vi "AVI_Tools.vi"() -> ()   [LabVIEW 2022 SP3]
uses:
  <vilib>/vision/Image Controls.llb/IMAQ Image.ctl
  <vilib>/vision/Avi.llb/IMAQ AVI2 Refnum.ctl
  <vilib>/vision/Avi.llb/IMAQ AVI2 Codec Path.ctl
panel:
  out "Array 2":i32[][](array[numeric])
  out "file name":string
  out "FinalImge":i32[](array[numeric])
  out "Crop Size":i32[](array[numeric])=[50, 60, 520, 360]
  in  "Tab Control":enum32{"Crop", "Output"}(tab)
  out "ref Fram":T1(plugin-control)
  in  "Crop":bool
  in  "Insertion Point":bool
  out "Output":T1(plugin-control)
  in  "Start SpliceFrame":i32=1000
  in  "#Frame":i32=260
  out "Frame":i32
  in  "Splice":u16(ring)=17 items=["Bmode CD"=17, "VPI"=26]
  out "CurrentSaveFile":string
  in  "Text Splice":u16(ring) items=["SelectText", "WT", "KO"]
  in  "Add text":string
  in  "DownSamp":u32=2
  in  "Group":i32=2
  in  "Scale":sgl
  in  "Codec Source":T2 items=["Default", "System", "Built in Vision"]
  in  "AVI save name":string
  out "Frames":u32[](array[numeric])
  out "Text Insertion Point":i32[](array[numeric])=[40, 20]
  in  "Enum":T3(ring)
  out "Array":T4(array[cluster])
  in  "Use Selected Files":bool
  in  "Listbox":i32[](listbox)
  in  "AviReadDirectory":path=path "D:/"
  in  "search pattern":string="*.avi"
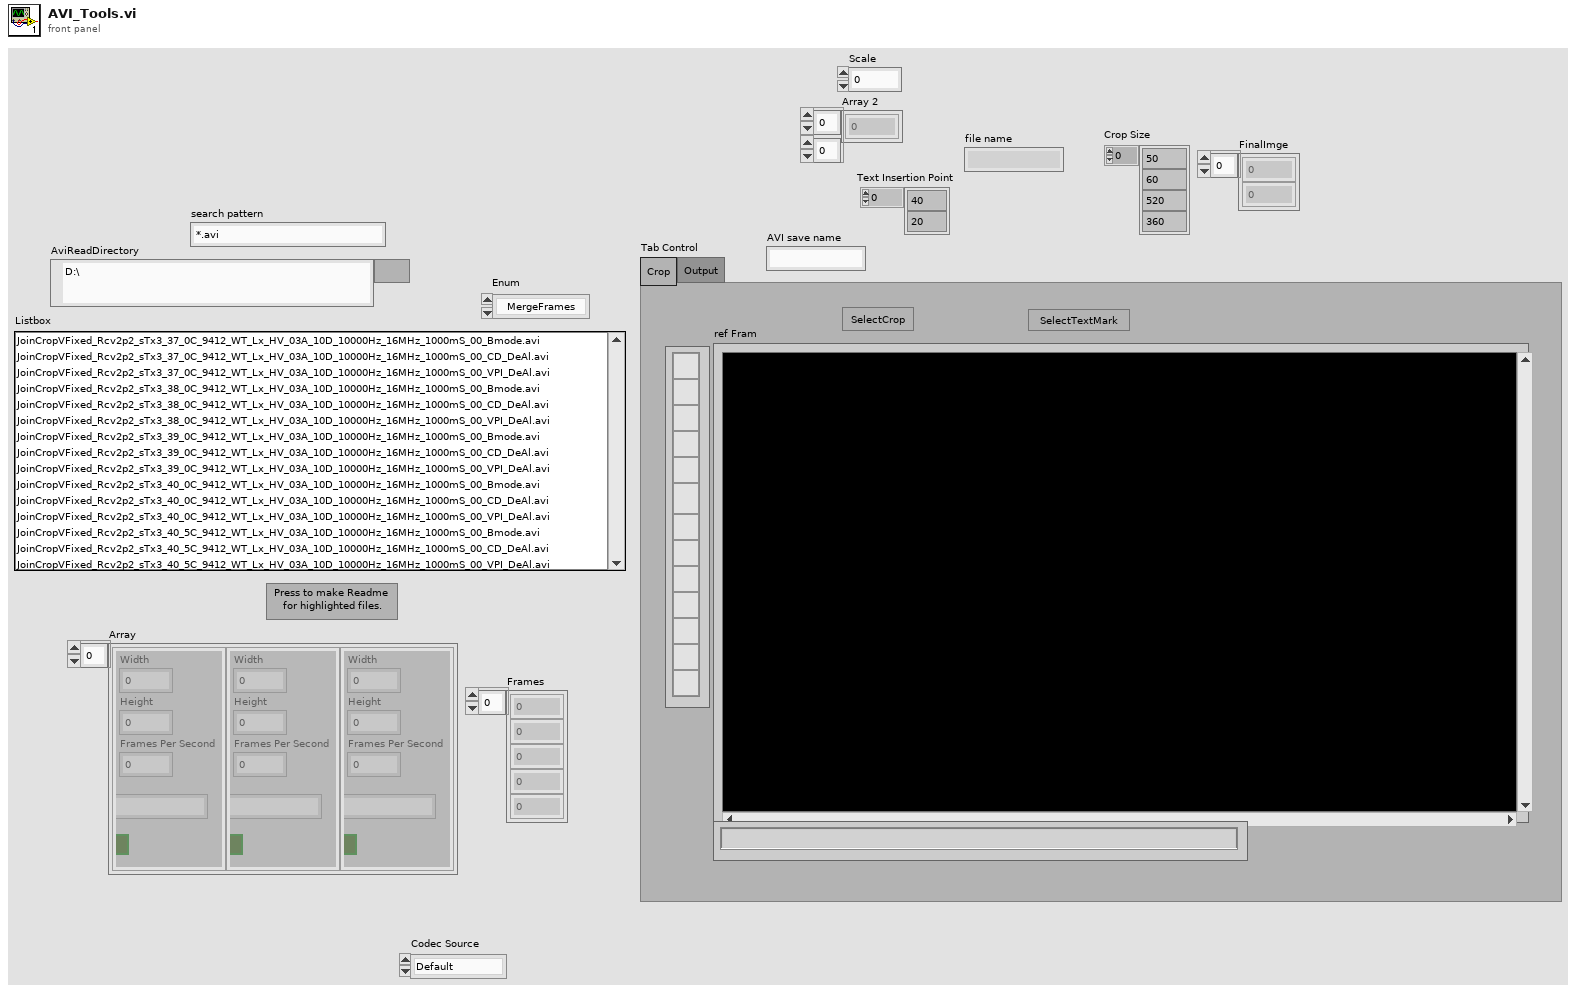
[diagram p1: front panel]
types:
  T1 = typedef "IMAQ Image.ctl" = refnum<image>
  T2 = typedef "IMAQ AVI2 Codec Path.ctl" = u32
  T3 = enum16{"MergeFrames", "Join AVI", "Crop", "OverlayText", "RescaleScale", "SpliceIn", "DownSample", "Extract"}
  T4 = cluster{"Width":u32, "Height":u32, "Frames Per Second":u32, "Codec":string, "Has Data":bool}[]
  T5 = typedef "IMAQ AVI2 Refnum.ctl" = refnum<k20>
  T6 = cluster{"Number of Frames":u32, "Frame Data":cluster{"Width":u32, "Height":u32, "Frames Per Second":u32, "Codec":string, "Has Data":bool}, "New Image":T1, "AVI Refnum":T5, "file name":string}
  T7 = typedef "Image Type" = u32
  T8 = cluster{"Width":u32, "Height":u32, "Frames Per Second":u32, "Codec":string, "Has Data":bool}
  T9 = cluster{"Desired Font (Application)":enum16{"User-specified Font", "Application Font", "System Font", "Dialog Font"}, "[User-specified Font]":cluster{"Font Name":string, "Size":i16, "Strikeout?":bool, "Italic?":bool, "Underline?":bool, "Outline?":bool, "Shadow?":bool, "Bold?":bool, "Rotation Angle":dbl}, "Horizontal Alignment":i16, "Vertical Alignment":i16}
  T10 = cluster{"Global Rectangle":i32[], "Contours":cluster{"Contour Type":u32, "ROI Type":u32, "Points":i32[]}[]}
  T11 = cluster{"Number of Frames":u32, "Frame Data":cluster{"Width":u32, "Height":u32, "Frames Per Second":u32, "Codec":string, "Has Data":bool}, "New Image":T1, "AVI Refnum":T5, "file name":string}[][]
  T12 = cluster{"Number of Frames":u32, "Frame Data":cluster{"Width":u32, "Height":u32, "Frames Per Second":u32, "Codec":string, "Has Data":bool}, "New Image":T1, "AVI Refnum":T5, "file name":string}[]
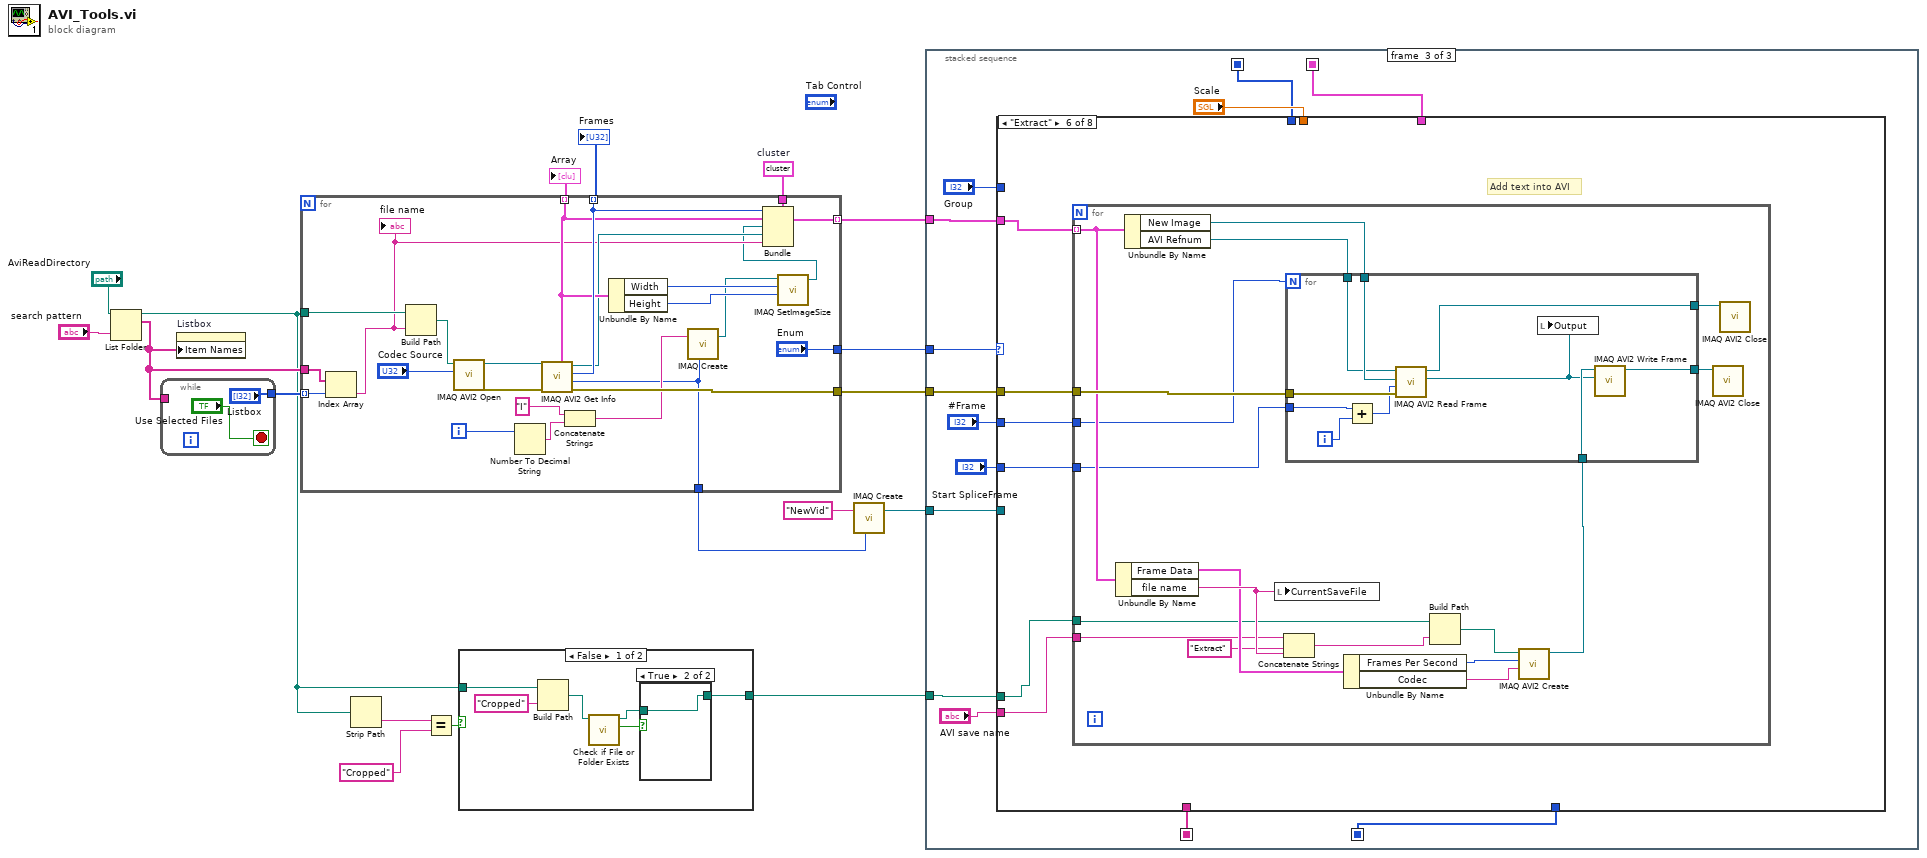
[diagram p0: block diagram]
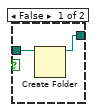
[diagram p2: hidden frame]
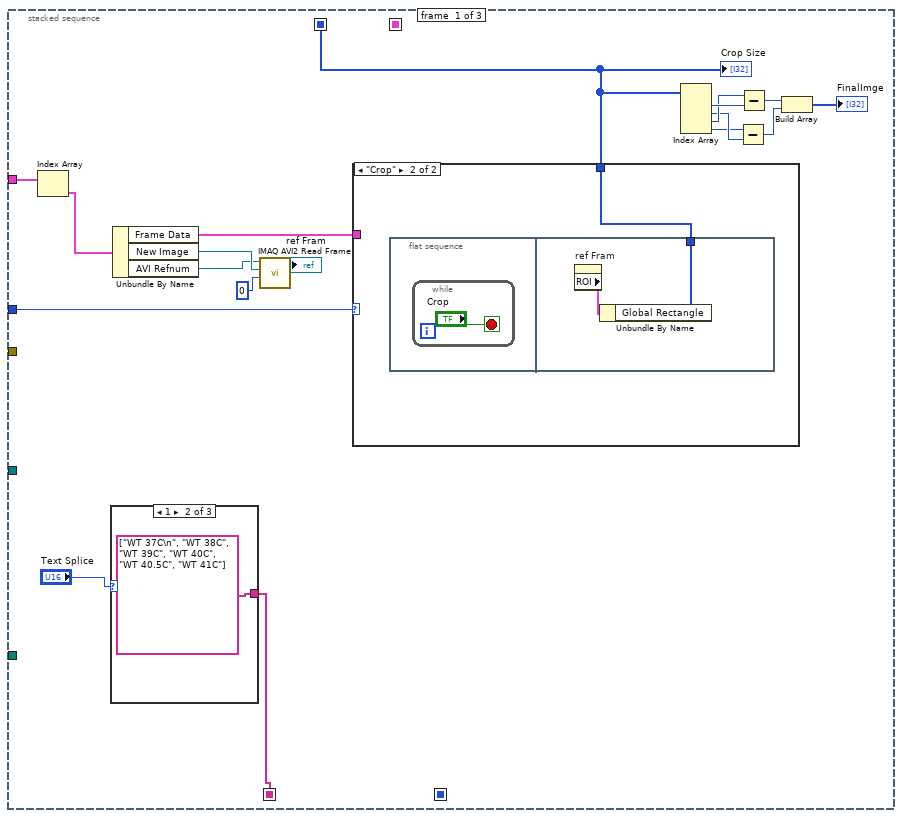
[diagram p4: hidden frame]
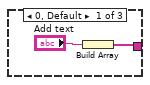
[diagram p5: hidden frame]
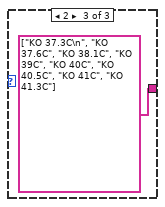
[diagram p6: hidden frame]
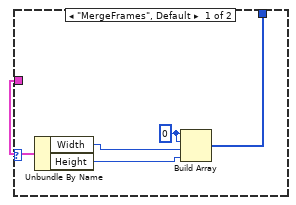
[diagram p7: hidden frame]
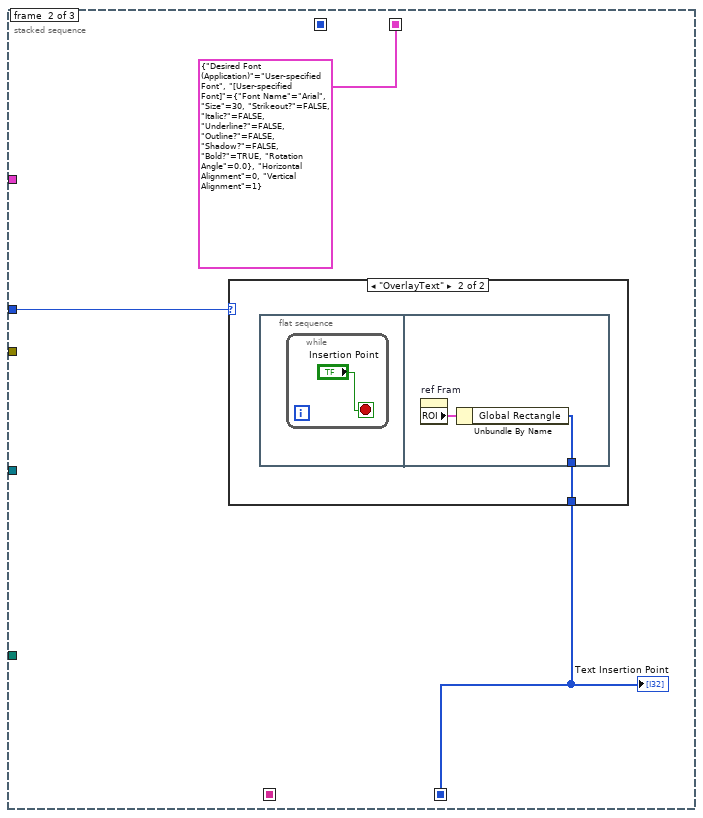
[diagram p8: hidden frame]
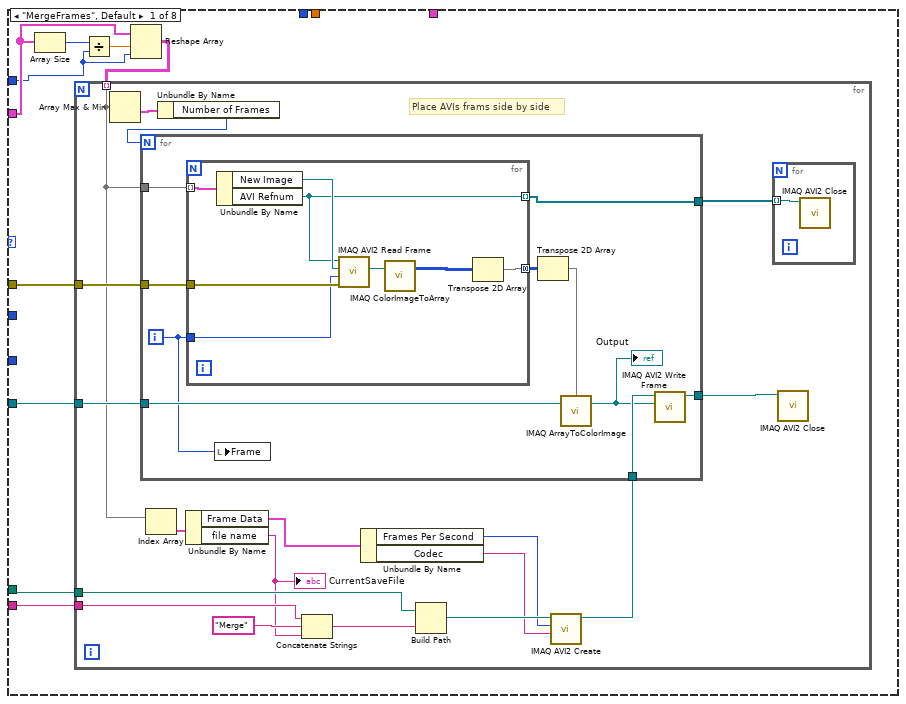
[diagram p10: hidden frame]
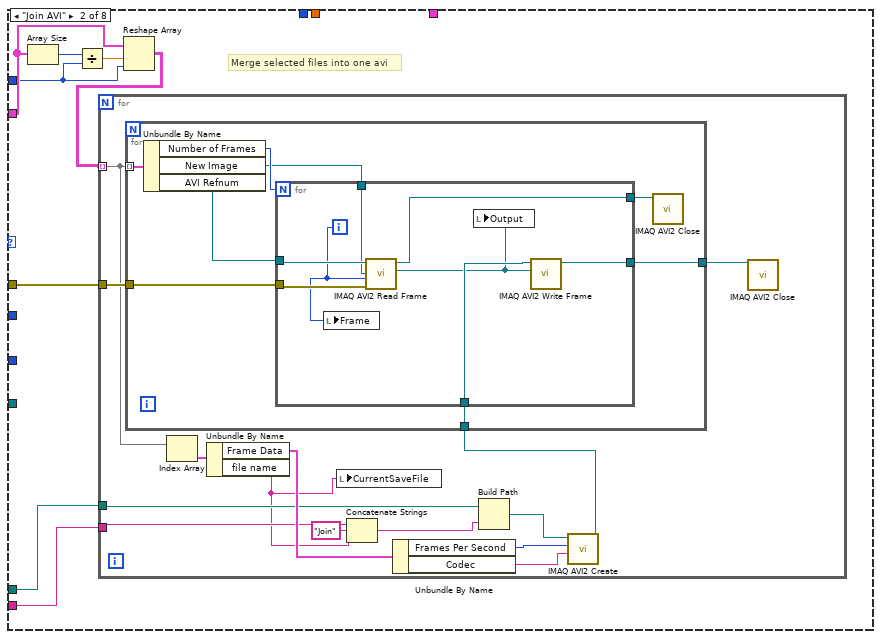
[diagram p11: hidden frame]
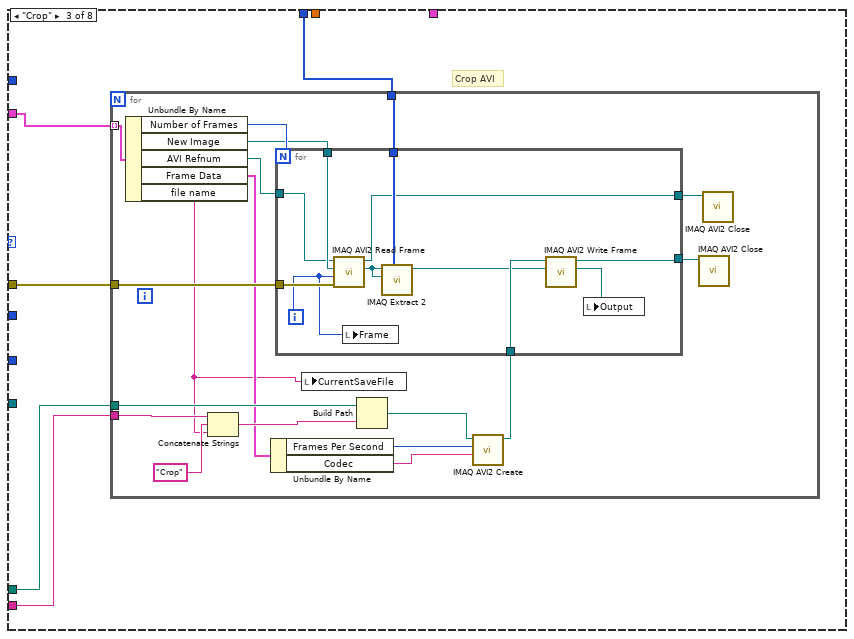
[diagram p12: hidden frame]
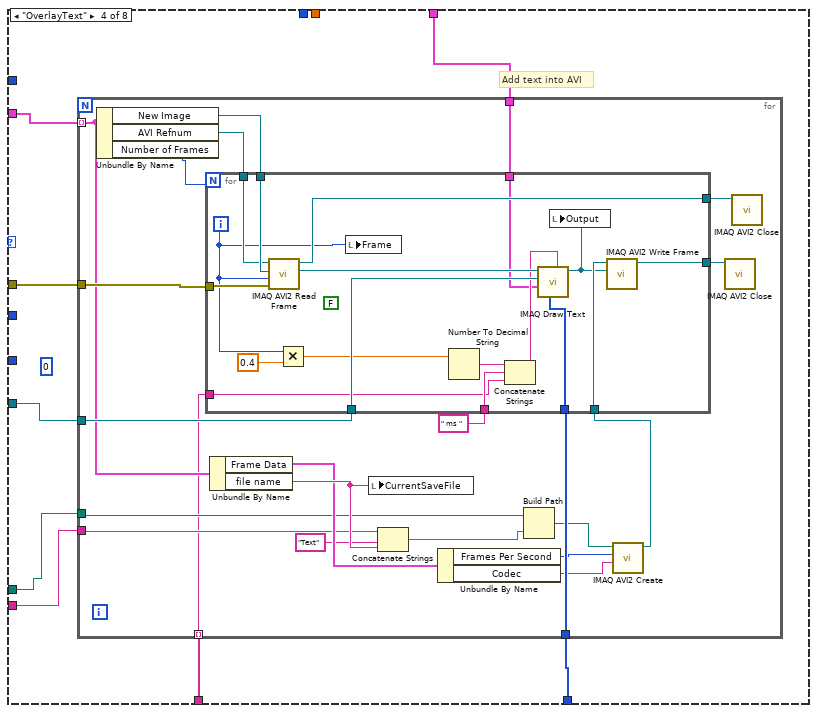
[diagram p13: hidden frame]
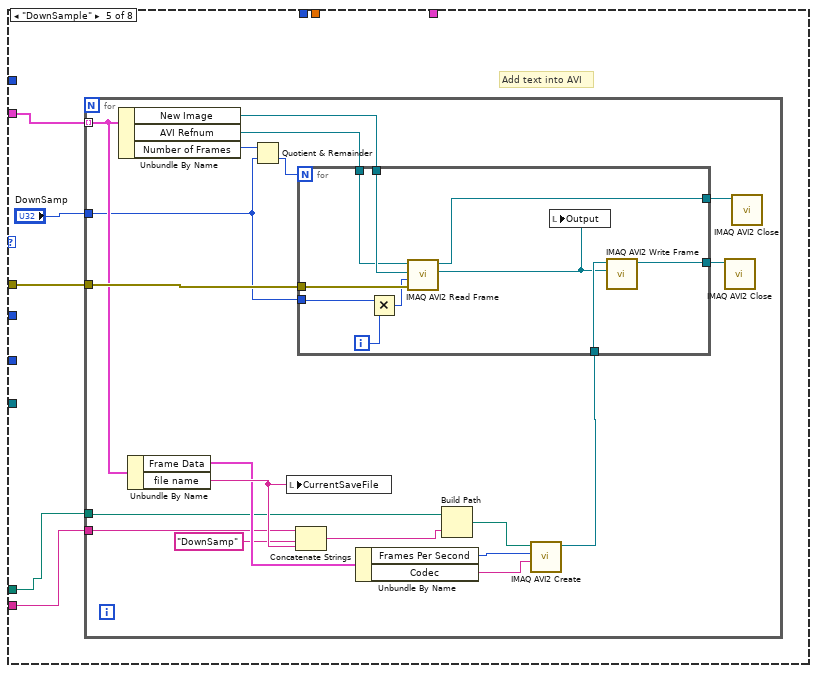
[diagram p14: hidden frame]
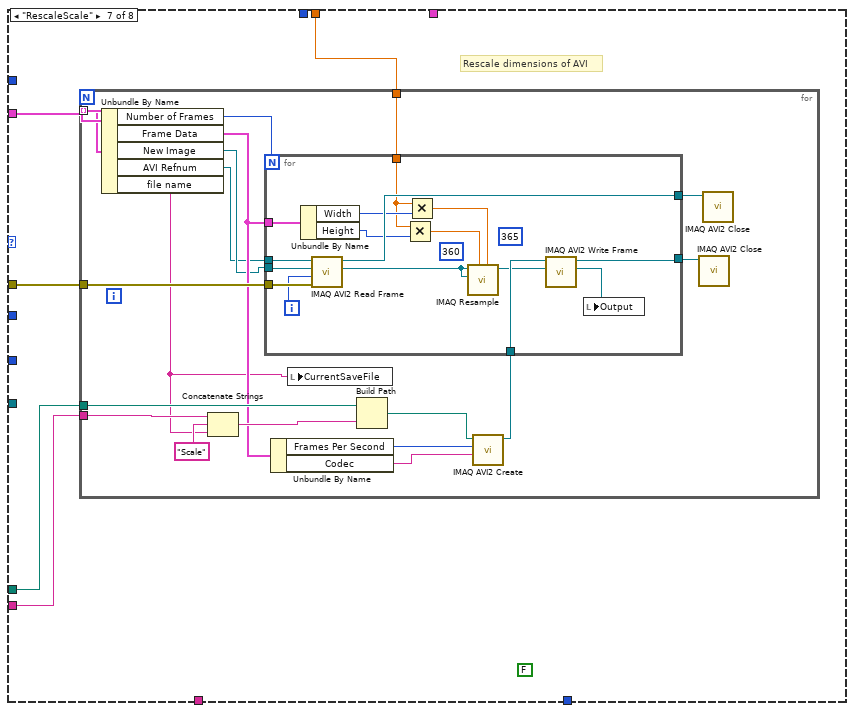
[diagram p15: hidden frame]
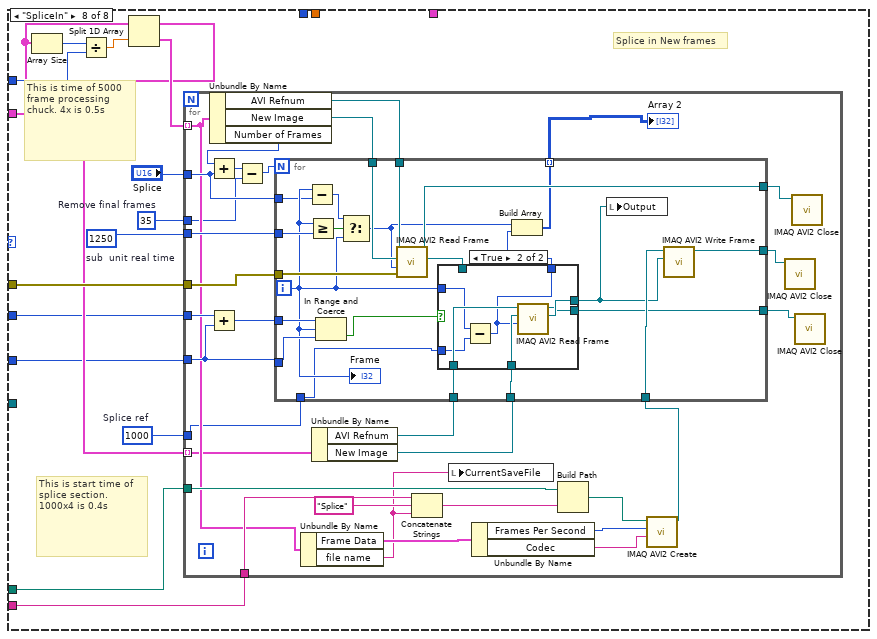
[diagram p16: hidden frame]
diagram:
  w2 = T6 {"Number of Frames"=0, "Frame Data"={"Width"=0, "Height"=0, "Frames Per Second"=0, "Codec"="", "Has Data"=FALSE}, "New Image"=refnum, "AVI Refnum"=refnum, "file name"=""}  # cluster
  n1 = List Folder(path="AviReadDirectory", pattern="search pattern") -> (path out=w7:path, filenames=w11:string[])  [unwired: 1 in, 3 out]
  n2 = while {
    tunnel: ["Listbox"] -> w13
    tunnel: w11 -> [_]
    stop <- "Use Selected Files" stop-if-true
  }
  n3 = property on="Listbox" class="LstBox (strict)"("Item Names"=w11) -> ()  [unwired: 2 in, 2 out]
  n4 = for {
    tunnel: [w42] -> w18
    tunnel: w13 -> [w39] mode=indexing
    tunnel: w11 -> [w38]
    tunnel: w7 -> [w37]
    tunnel: [w31] -> w10
    tunnel: [w28] -> w12 mode=indexing
    tunnel: [w29] -> w9 mode=indexing
    tunnel: [w25] -> w3 mode=indexing
    tunnel: w2 -> [w24]
    tunnel: ["Enum"] -> w1
    i -> [w35]
    n5 = Index Array(array=w38, index=w39) -> (element=w23:string)
    "file name" <- w23
    n6 = Build Path(base path=w37, name or relative path=w23) -> (appended path=w36:path)
    n7 = call "IMAQ AVI2 Open"("Codec Source"="Codec Source", "AVI File Path"=w36) -> ("error out"=w43:errorcluster, "AVI Refnum"=w44:T5)  [unwired: 8 in]
    n8 = Number To Decimal String(number=w35) -> (decimal integer string=w33:string)  [unwired: 1 in]
    n9 = call "IMAQ AVI2 Get Info"("error in (no error)"=w43, "AVI Refnum"=w44) -> ("error out"=w42:errorcluster, "Image Type"=w31:T7, "Number of Frames"=w29:u32, "AVI Refnum (duplicate)"=w26:T5, "Frame Data"=w28:T8)  [unwired: 5 out]
    n10 = Concatenate Strings("I" ("Image Name"), w33) -> (w32:string)
    n11 = Unbundle By Name(w28) -> ("Width"=w41:u32, "Height"=w40:u32)
    n12 = call "IMAQ Create"("Image Name"=w32, "Image Type"=w31) -> ("New Image"=w27:T1)  [unwired: 2 in, 2 out]
    n13 = call "IMAQ SetImageSize"("Y Resolution"=w40, "X Resolution"=w41, "Image"=w27) -> ("Image Out"=w22:T1)  [unwired: 2 in, 1 out]
    n14 = Bundle(cluster=w24, "Number of Frames"=w29, "Frame Data"=w28, "New Image"=w22, "AVI Refnum"=w26, "file name"=w23) -> (w25:T6)
  }
  "Array" <- w12
  "Frames" <- w9
  n15 = Strip Path(path=w7) -> (name=w6:string)  [unwired: 1 out]
  n16 = Equal?(x=w6, y="Cropped" ("name or relative path")) -> (x = y?=w4:bool)
  n17 = case shown="False" w4 {
    tunnel: [w45 w54] -> w8
    tunnel: w7 -> [w49 w54]
    frame False {
      n18 = Build Path(base path=w49, name or relative path="Cropped") -> (appended path=w46:path)
      n19 = call <vilib>:"Check if File or Folder Exists.vi"("path"=w46) -> ("file or folder exists?"=w47:bool, "dup path"=w48:path)  [unwired: 8 in, 1 out]
      n20 = case shown="True" w47 {
        tunnel: w48 -> [w52 w53]
        tunnel: [w51 w53] -> w45
        frame False {
          n21 = Create Folder(path (use dialog)=w52) -> (created path=w51:path)  [unwired: 2 in, 2 out]
        }
        frame True {
        }
      }
    }
    frame True {
    }
  }
  n22 = call "IMAQ Create"("Image Name"="NewVid", "Image Type"=w10) -> ("New Image"=w14:T1)  [unwired: 2 in, 2 out]
  n23 = stacked-sequence {
    seq-local: [w65 _ _] -> [_ _ w103]
    seq-local: [_ w87 _] -> [_ _ w102]
    seq-local: [_ T9 {"Desired Font (Application)"=enum."User-specified Font", "[User-specified Font]"={"Font Name"="Arial", "Size"=30, "Strikeout?"=FALSE, "Italic?"=FALSE, "Underline?"=FALSE, "Outline?"=FALSE, "Shadow?"=FALSE, "Bold?"=TRUE, "Rotation Angle"=0.0}, "Horizontal Alignment"=0, "Vertical Alignment"=1} ("Font, Size & Style") _] -> [_ _ w101]
    seq-local: [w57 _ _] -> [_ _ w96]
    tunnel: w18 -> [_ _ w106]
    tunnel: w14 -> [_ _ w105]
    tunnel: w8 -> [_ _ w100]
    tunnel: w3 -> [w62 _ w98]
    tunnel: w1 -> [w55 w86 w95]
    frame #0 {
      n24 = Index Array(array=w62) -> (element=w61:T6)  [unwired: 1 in]
      n25 = case shown="1" "Text Splice" {
        tunnel: [w74 string[] ["WT 37C\n", "WT 38C", "WT 39C", "WT 40C", "WT 40.5C", "WT 41C"] string[] ["KO 37.3C\n", "KO 37.6C", "KO 38.1C", "KO 39C", "KO 40C", "KO 40.5C", "KO 41C", "KO 41.3C"]] -> w57
        frame 0, Default {
          n26 = Build Array("Add text") -> (w74:string[])
        }
        frame 1 {
        }
        frame 2 {
        }
      }
      n27 = Unbundle By Name(w61) -> ("Frame Data"=w60:T8, "New Image"=w59:T1, "AVI Refnum"=w58:T5)
      n28 = call "IMAQ AVI2 Read Frame"("Frame Number"=u32 0, "Image"=w59, "AVI Refnum"=w58) -> ("Image Out"=→"ref Fram":T1)  [unwired: 6 in, 2 out]
      n29 = case shown="\"Crop\"" w55 {
        tunnel: [w78 w82] -> w65
        tunnel: w60 -> [w77 _]
        frame "MergeFrames", Default {
          w79 = u32 0 ("element")
          n30 = Unbundle By Name(w77) -> ("Width"=w81:u32, "Height"=w80:u32)
          n31 = Build Array(w79, w79, w81, w80) -> (w78:u32[])
        }
        frame "Crop" {
          n32 = flat-sequence {
            tunnel: [w84] -> w82
            frame #0 {
              n33 = while {
                stop <- "Crop" stop-if-true
              }
            }
            frame #1 {
              n34 = property on="ref Fram" class="ImageControl"() -> ("ROI"=w85:T10)  [unwired: 2 in, 2 out]
              n35 = Unbundle By Name(w85) -> ("Global Rectangle"=w84:i32[])
            }
          }
        }
      }
      "Crop Size" <- w65
      n36 = Index Array(array=w65) -> (element #1=w69:u32, element #2=w67:u32, element #3=w68:u32, element #4=w66:u32)  [unwired: 4 in]
      n37 = Subtract(x=w66, y=w67) -> (x-y=w71:u32)
      n38 = Subtract(x=w68, y=w69) -> (x-y=w70:u32)
      n39 = Build Array(w70, w71) -> (→"FinalImge":u32[])
    }
    frame #1 {
      n40 = case shown="\"OverlayText\"" w86 {
        tunnel: [_ w89] -> w87
        frame "MergeFrames", Default {
        }
        frame "OverlayText" {
          n41 = flat-sequence {
            tunnel: [w91] -> w89
            frame #0 {
              n42 = while {
                stop <- "Insertion Point" stop-if-true
              }
            }
            frame #1 {
              n43 = property on="ref Fram" class="ImageControl"() -> ("ROI"=w92:T10)  [unwired: 2 in, 2 out]
              n44 = Unbundle By Name(w92) -> ("Global Rectangle"=w91:i32[])
            }
          }
        }
      }
      "Text Insertion Point" <- w87
    }
    frame #2 {
      n45 = case shown="\"Extract\"" w95 {
        tunnel: w106 -> [w115 w160 w195 w232 w277 w312 w345 w394]
        tunnel: w105 -> [w114 _ _ w231 _ _ _ _]
        tunnel: w103 -> [_ _ w194 _ _ _ _ _]
        tunnel: w101 -> [_ _ _ w230 _ _ _ _]
        tunnel: w102 -> [_ _ _ w226 _ _ _ _]
        tunnel: "Scale" -> [_ _ _ _ _ _ w342 _]
        tunnel: w100 -> [w113 w155 w193 w227 w274 w309 w344 w392]
        tunnel: "AVI save name" -> [w112 w156 w192 w228 w275 w310 w343 w393]
        tunnel: w98 -> [w109 w157 w191 w229 w276 w311 w341 w388]
        tunnel: "Group" -> [w108 w153 _ _ _ _ _ w390]
        tunnel: w96 -> [_ _ _ w225 _ _ _ _]
        tunnel: "Start SpliceFrame" -> [_ _ _ _ _ w307 _ w381]
        tunnel: "#Frame" -> [_ _ _ _ _ w308 _ w380]
        frame "MergeFrames", Default {
          n46 = Array Size(array=w109) -> (size(s)=w111:i32)
          n47 = Divide(x=w111, y=w108) -> (x/y=w110:dbl)
          n48 = Reshape Array(w109, w110, w108) -> (w107:T11)
          n49 = for {
            tunnel: w115 -> [w133]
            tunnel: w114 -> [w132]
            tunnel: w113 -> [w124]
            tunnel: w112 -> [w123]
            tunnel: w107 -> [w116] mode=indexing
            # "Place AVIs frams side by side"
            n50 = Array Max & Min(array=w116) -> (min value=w118:T6)  [unwired: 3 out]
            n51 = Index Array(array=w116) -> (element=w121:T6)  [unwired: 1 in]
            n52 = Unbundle By Name(w118) -> ("Number of Frames"=w117:u32)
            n53 = Unbundle By Name(w121) -> ("Frame Data"=w119:T8, "file name"=w120:string)
            "CurrentSaveFile" <- w120
            n54 = Concatenate Strings(w123, "Merge" ("string"), w120) -> (w129:string)
            n55 = Unbundle By Name(w119) -> ("Frames Per Second"=w126:u32, "Codec"=w127:string)
            n56 = Build Path(base path=w124, name or relative path=w129) -> (appended path=w128:path)
            n57 = call "IMAQ AVI2 Create"("Codec"=w127, "Frames Per Second"=w126, "AVI Path"=w128) -> ("AVI Refnum"=w125:T5)  [unwired: 7 in, 1 out]
            n58 = for {
              N: w117 -> [_]
              tunnel: w133 -> [w144]
              tunnel: w125 -> [w143]
              tunnel: [w141] -> w130
              tunnel: w132 -> [w140]
              tunnel: [w135] -> w131
              tunnel: w116 -> [w136]
              i -> [w138]
              n59 = for {
                tunnel: w144 -> [w152]
                tunnel: [w148] -> w139 mode=concatenating
                tunnel: w138 -> [w151]
                tunnel: w136 -> [w147] mode=indexing
                tunnel: [w145] -> w135 mode=indexing
                n60 = Unbundle By Name(w147) -> ("New Image"=w146:T1, "AVI Refnum"=w145:T5)
                n61 = call "IMAQ AVI2 Read Frame"("error in (no error)"=w152, "Frame Number"=w151, "Image"=w146, "AVI Refnum"=w145) -> ("Image Out"=w150:T1)  [unwired: 5 in, 2 out]
                n62 = call "IMAQ ColorImageToArray"("Image"=w150) -> ("Image Pixels (U32)"=w149:u32[][])  [unwired: 3 in, 2 out]
                n63 = Transpose 2D Array(2D array=w149) -> (transposed array=w148:u32[][])
              }
              n64 = local write "Frame"(w138) -> ()
              n65 = Transpose 2D Array(2D array=w139) -> (transposed array=w137:u32[][])
              n66 = call "IMAQ ArrayToColorImage"("Image Pixels (U32)"=w137, "Image"=w140) -> ("Image Out"=w142:T1)  [unwired: 3 in, 1 out]
              "Output" <- w142
              n67 = call "IMAQ AVI2 Write Frame"("Image"=w142, "AVI Refnum"=w143) -> ("AVI Refnum (duplicate)"=w141:T5)  [unwired: 7 in, 2 out]
            }
            n68 = for {
              tunnel: w131 -> [w134] mode=indexing
              n69 = call "IMAQ AVI2 Close"("AVI Refnum"=w134) -> ()  [unwired: 10 in, 1 out]
            }
            n70 = call "IMAQ AVI2 Close"("AVI Refnum"=w130) -> ()  [unwired: 10 in, 1 out]
          }
        }
        frame "Join AVI" {
          # "Merge selected files into one avi"
          n71 = Array Size(array=w157) -> (size(s)=w159:i32)
          n72 = Divide(x=w159, y=w153) -> (x/y=w154:dbl)
          n73 = Reshape Array(w157, w154, w153) -> (w158:T11)
          n74 = for {
            tunnel: w160 -> [w174]
            tunnel: w158 -> [w162] mode=indexing
            tunnel: w156 -> [w166]
            tunnel: w155 -> [w164]
            n75 = Index Array(array=w162) -> (element=w171:T6)  [unwired: 1 in]
            n76 = Unbundle By Name(w171) -> ("Frame Data"=w172:T8, "file name"=w161:string)
            n77 = local write "CurrentSaveFile"(w161) -> ()
            n78 = Concatenate Strings(w166, "Join" ("string"), w161) -> (w167:string)
            n79 = Unbundle By Name(w172) -> ("Frames Per Second"=w170:u32, "Codec"=w169:string)
            n80 = Build Path(base path=w164, name or relative path=w167) -> (appended path=w168:path)
            n81 = call "IMAQ AVI2 Create"("Codec"=w169, "Frames Per Second"=w170, "AVI Path"=w168) -> ("AVI Refnum"=w163:T5)  [unwired: 7 in, 1 out]
            n82 = for {
              tunnel: w174 -> [w182]
              tunnel: w163 -> [w180]
              tunnel: [w181] -> w173
              tunnel: w162 -> [w178] mode=indexing
              n83 = Unbundle By Name(w178) -> ("Number of Frames"=w177:u32, "New Image"=w175:T1, "AVI Refnum"=w176:T5)
              n84 = for {
                N: w177 -> [_]
                tunnel: w182 -> [w187]
                tunnel: [w190] -> w181
                tunnel: [w189] -> w179
                tunnel: w176 -> [w188]
                tunnel: w180 -> [w186]
                tunnel: w175 -> [w183]
                i -> [w184]
                n85 = local write "Frame"(w184) -> ()
                n86 = call "IMAQ AVI2 Read Frame"("error in (no error)"=w187, "Frame Number"=w184, "Image"=w183, "AVI Refnum"=w188) -> ("Image Out"=w185:T1, "AVI Refnum (duplicate)"=w189:T5)  [unwired: 5 in, 1 out]
                n87 = local write "Output"(w185) -> ()
                n88 = call "IMAQ AVI2 Write Frame"("Image"=w185, "AVI Refnum"=w186) -> ("AVI Refnum (duplicate)"=w190:T5)  [unwired: 7 in, 2 out]
              }
              n89 = call "IMAQ AVI2 Close"("AVI Refnum"=w179) -> ()  [unwired: 10 in, 1 out]
            }
            n90 = call "IMAQ AVI2 Close"("AVI Refnum"=w173) -> ()  [unwired: 10 in, 1 out]
          }
        }
        frame "Crop" {
          # "Crop AVI"
          n91 = for {
            tunnel: w195 -> [w213]
            tunnel: w194 -> [w212]
            tunnel: w193 -> [w208]
            tunnel: w192 -> [w204]
            tunnel: w191 -> [w201] mode=indexing
            n92 = Unbundle By Name(w201) -> ("Number of Frames"=w200:u32, "New Image"=w199:T1, "AVI Refnum"=w198:T5, "Frame Data"=w197:T8, "file name"=w196:string)
            n93 = Concatenate Strings(w204, "Crop" ("string"), w196) -> (w207:string)
            n94 = Unbundle By Name(w197) -> ("Frames Per Second"=w211:u32, "Codec"=w210:string)
            n95 = local write "CurrentSaveFile"(w196) -> ()
            n96 = Build Path(base path=w208, name or relative path=w207) -> (appended path=w209:path)
            n97 = call "IMAQ AVI2 Create"("Codec"=w210, "Frames Per Second"=w211, "AVI Path"=w209) -> ("AVI Refnum"=w206:T5)  [unwired: 7 in, 1 out]
            n98 = for {
              N: w200 -> [_]
              tunnel: w213 -> [w224]
              tunnel: w212 -> [w222]
              tunnel: w206 -> [w221]
              tunnel: [w218] -> w205
              tunnel: [w217] -> w203
              tunnel: w199 -> [w215]
              tunnel: w198 -> [w214]
              i -> [w216]
              n99 = call "IMAQ AVI2 Read Frame"("error in (no error)"=w224, "Frame Number"=w216, "Image"=w215, "AVI Refnum"=w214) -> ("Image Out"=w223:T1, "AVI Refnum (duplicate)"=w217:T5)  [unwired: 5 in, 1 out]
              n100 = local write "Frame"(w216) -> ()
              n101 = call "IMAQ Extract 2"("Optional Rectangle"=w222, "Image Dst"=w223, "Image Src"=w223) -> ("Image Dst Out"=w220:T1)  [unwired: 7 in, 1 out]
              n102 = call "IMAQ AVI2 Write Frame"("Image"=w220, "AVI Refnum"=w221) -> ("Image Out (duplicate)"=w219:T1, "AVI Refnum (duplicate)"=w218:T5)  [unwired: 7 in, 1 out]
              n103 = local write "Output"(w219) -> ()
            }
            n104 = call "IMAQ AVI2 Close"("AVI Refnum"=w205) -> ()  [unwired: 10 in, 1 out]
            n105 = call "IMAQ AVI2 Close"("AVI Refnum"=w203) -> ()  [unwired: 10 in, 1 out]
          }
        }
        frame "OverlayText" {
          (unwired) 0
          # "Add text into AVI"
          n106 = for {
            tunnel: w232 -> [w254]
            tunnel: w231 -> [w253]
            tunnel: w230 -> [w252]
            tunnel: w226 -> [w251]
            tunnel: w229 -> [w234] mode=indexing
            tunnel: w228 -> [w238]
            tunnel: w227 -> [w236]
            tunnel: w225 -> [w233] mode=indexing
            n107 = Unbundle By Name(w234) -> ("New Image"=w247:T1, "AVI Refnum"=w246:T5, "Number of Frames"=w245:u32)
            n108 = Unbundle By Name(w234) -> ("Frame Data"=w243:T8, "file name"=w244:string)
            n109 = local write "CurrentSaveFile"(w244) -> ()
            n110 = Concatenate Strings(w238, "Text" ("string"), w244) -> (w239:string)
            n111 = Unbundle By Name(w243) -> ("Frames Per Second"=w242:u32, "Codec"=w241:string)
            n112 = Build Path(base path=w236, name or relative path=w239) -> (appended path=w240:path)
            n113 = call "IMAQ AVI2 Create"("Codec"=w241, "Frames Per Second"=w242, "AVI Path"=w240) -> ("AVI Refnum"=w235:T5)  [unwired: 7 in, 1 out]
            n114 = for {
              N: w245 -> [_]
              tunnel: w254 -> [w266]
              tunnel: w253 -> [w268]
              tunnel: [w271] -> w250
              tunnel: [w270] -> w249
              tunnel: w235 -> [w269]
              tunnel: w252 -> [w263]
              tunnel: w251 -> [w262]
              tunnel: " ms " ("string") -> [w261]
              tunnel: w247 -> [w260]
              tunnel: w246 -> [w259]
              tunnel: w233 -> [w255]
              i -> [w258]
              (unwired) FALSE
              n115 = call "IMAQ AVI2 Read Frame"("error in (no error)"=w266, "Frame Number"=w258, "Image"=w260, "AVI Refnum"=w259) -> ("Image Out"=w272:T1, "AVI Refnum (duplicate)"=w270:T5)  [unwired: 5 in, 1 out]
              n116 = Multiply(x=w258, y=0.4) -> (x*y=w256:dbl)
              n117 = local write "Frame"(w258) -> ()
              n118 = Number To Decimal String(number=w256) -> (decimal integer string=w265:string)  [unwired: 1 in]
              n119 = Concatenate Strings(w265, w261, w255) -> (w264:string)
              n120 = call "IMAQ Draw Text"("String"=w264, "Insertion Point"=w262, "Font, Size & Style"=w263, "Image Dst"=w268, "Image Src"=w272) -> ("Image Dst Out"=w267:T1)  [unwired: 3 in, 3 out]
              n121 = local write "Output"(w267) -> ()
              n122 = call "IMAQ AVI2 Write Frame"("Image"=w267, "AVI Refnum"=w269) -> ("AVI Refnum (duplicate)"=w271:T5)  [unwired: 7 in, 2 out]
            }
            n123 = call "IMAQ AVI2 Close"("AVI Refnum"=w250) -> ()  [unwired: 10 in, 1 out]
            n124 = call "IMAQ AVI2 Close"("AVI Refnum"=w249) -> ()  [unwired: 10 in, 1 out]
          }
        }
        frame "DownSample" {
          # "Add text into AVI"
          n125 = for {
            tunnel: w277 -> [w296]
            tunnel: w276 -> [w281] mode=indexing
            tunnel: w275 -> [w285]
            tunnel: w274 -> [w283]
            tunnel: "DownSamp" -> [w278]
            n126 = Unbundle By Name(w281) -> ("New Image"=w293:T1, "AVI Refnum"=w292:T5, "Number of Frames"=w280:u32)
            n127 = Unbundle By Name(w281) -> ("Frame Data"=w290:T8, "file name"=w291:string)
            n128 = Quotient & Remainder(x=w280, y=w278) -> (floor(x/y)=w279:u32)  [unwired: 1 out]
            n129 = local write "CurrentSaveFile"(w291) -> ()
            n130 = Concatenate Strings(w285, "DownSamp" ("string"), w291) -> (w286:string)
            n131 = Unbundle By Name(w290) -> ("Frames Per Second"=w289:u32, "Codec"=w288:string)
            n132 = Build Path(base path=w283, name or relative path=w286) -> (appended path=w287:path)
            n133 = call "IMAQ AVI2 Create"("Codec"=w288, "Frames Per Second"=w289, "AVI Path"=w287) -> ("AVI Refnum"=w282:T5)  [unwired: 7 in, 1 out]
            n134 = for {
              N: w279 -> [_]
              tunnel: w296 -> [w303]
              tunnel: [w306] -> w295
              tunnel: [w305] -> w294
              tunnel: w282 -> [w304]
              tunnel: w293 -> [w302]
              tunnel: w292 -> [w301]
              tunnel: w278 -> [w299]
              i -> [w300]
              n135 = Multiply(x=w299, y=w300) -> (x*y=w298:u32)
              n136 = call "IMAQ AVI2 Read Frame"("error in (no error)"=w303, "Frame Number"=w298, "Image"=w302, "AVI Refnum"=w301) -> ("Image Out"=w297:T1, "AVI Refnum (duplicate)"=w305:T5)  [unwired: 5 in, 1 out]
              n137 = local write "Output"(w297) -> ()
              n138 = call "IMAQ AVI2 Write Frame"("Image"=w297, "AVI Refnum"=w304) -> ("AVI Refnum (duplicate)"=w306:T5)  [unwired: 7 in, 2 out]
            }
            n139 = call "IMAQ AVI2 Close"("AVI Refnum"=w295) -> ()  [unwired: 10 in, 1 out]
            n140 = call "IMAQ AVI2 Close"("AVI Refnum"=w294) -> ()  [unwired: 10 in, 1 out]
          }
        }
        frame "Extract" {
          # "Add text into AVI"
          n141 = for {
            tunnel: w312 -> [w330]
            tunnel: w311 -> [w315] mode=indexing
            tunnel: w310 -> [w319]
            tunnel: w309 -> [w317]
            tunnel: w308 -> [w314]
            tunnel: w307 -> [w313]
            n142 = Unbundle By Name(w315) -> ("Frame Data"=w324:T8, "file name"=w325:string)
            n143 = Unbundle By Name(w315) -> ("New Image"=w327:T1, "AVI Refnum"=w326:T5)
            n144 = local write "CurrentSaveFile"(w325) -> ()
            n145 = Concatenate Strings(w319, "Extract" ("string"), w325) -> (w320:string)
            n146 = Unbundle By Name(w324) -> ("Frames Per Second"=w323:u32, "Codec"=w322:string)
            n147 = Build Path(base path=w317, name or relative path=w320) -> (appended path=w321:path)
            n148 = call "IMAQ AVI2 Create"("Codec"=w322, "Frames Per Second"=w323, "AVI Path"=w321) -> ("AVI Refnum"=w316:T5)  [unwired: 7 in, 1 out]
            n149 = for {
              N: w314 -> [_]
              tunnel: w330 -> [w337]
              tunnel: [w340] -> w329
              tunnel: [w339] -> w328
              tunnel: w316 -> [w338]
              tunnel: w327 -> [w336]
              tunnel: w326 -> [w335]
              tunnel: w313 -> [w331]
              i -> [w333]
              n150 = Add(x=w331, y=w333) -> (x+y=w332:i32)
              n151 = call "IMAQ AVI2 Read Frame"("error in (no error)"=w337, "Frame Number"=w332, "Image"=w336, "AVI Refnum"=w335) -> ("Image Out"=w334:T1, "AVI Refnum (duplicate)"=w339:T5)  [unwired: 5 in, 1 out]
              n152 = local write "Output"(w334) -> ()
              n153 = call "IMAQ AVI2 Write Frame"("Image"=w334, "AVI Refnum"=w338) -> ("AVI Refnum (duplicate)"=w340:T5)  [unwired: 7 in, 2 out]
            }
            n154 = call "IMAQ AVI2 Close"("AVI Refnum"=w329) -> ()  [unwired: 10 in, 1 out]
            n155 = call "IMAQ AVI2 Close"("AVI Refnum"=w328) -> ()  [unwired: 10 in, 1 out]
          }
        }
        frame "RescaleScale" {
          (unwired) FALSE
          # "Rescale dimensions of AVI"
          n156 = for {
            tunnel: w345 -> [w363]
            tunnel: w344 -> [w359]
            tunnel: w343 -> [w355]
            tunnel: w342 -> [w353]
            tunnel: w341 -> [w352] mode=indexing
            n157 = Unbundle By Name(w352) -> ("Number of Frames"=w351:u32, "Frame Data"=w350:T8, "New Image"=w349:T1, "AVI Refnum"=w348:T5, "file name"=w346:string)
            n158 = Concatenate Strings(w355, "Scale" ("string"), w346) -> (w358:string)
            n159 = Unbundle By Name(w350) -> ("Frames Per Second"=w362:u32, "Codec"=w361:string)
            n160 = local write "CurrentSaveFile"(w346) -> ()
            n161 = Build Path(base path=w359, name or relative path=w358) -> (appended path=w360:path)
            n162 = call "IMAQ AVI2 Create"("Codec"=w361, "Frames Per Second"=w362, "AVI Path"=w360) -> ("AVI Refnum"=w357:T5)  [unwired: 7 in, 1 out]
            n163 = for {
              N: w351 -> [_]
              tunnel: w348 -> [w379]
              tunnel: w363 -> [w378]
              tunnel: w349 -> [w377]
              tunnel: w357 -> [w376]
              tunnel: [w374] -> w356
              tunnel: [w373] -> w354
              tunnel: w353 -> [w365]
              tunnel: w350 -> [w364]
              i -> [w372]
              (unwired) 365 ("X Resolution")
              (unwired) 360 ("Y Resolution")
              n164 = Unbundle By Name(w364) -> ("Width"=w369:u32, "Height"=w368:u32)
              n165 = call "IMAQ AVI2 Read Frame"("error in (no error)"=w378, "Frame Number"=w372, "Image"=w377, "AVI Refnum"=w379) -> ("Image Out"=w367:T1, "AVI Refnum (duplicate)"=w373:T5)  [unwired: 5 in, 1 out]
              n166 = Multiply(x=w365, y=w368) -> (x*y=w370:sgl)
              n167 = Multiply(x=w365, y=w369) -> (x*y=w371:sgl)
              n168 = call "IMAQ Resample"("X Resolution"=w371, "Y Resolution"=w370, "Image Dst"=w367, "Image Src"=w367) -> ("Image Dst Out"=w366:T1)  [unwired: 6 in, 1 out]
              n169 = call "IMAQ AVI2 Write Frame"("Image"=w366, "AVI Refnum"=w376) -> ("Image Out (duplicate)"=w375:T1, "AVI Refnum (duplicate)"=w374:T5)  [unwired: 7 in, 1 out]
              n170 = local write "Output"(w375) -> ()
            }
            n171 = call "IMAQ AVI2 Close"("AVI Refnum"=w356) -> ()  [unwired: 10 in, 1 out]
            n172 = call "IMAQ AVI2 Close"("AVI Refnum"=w354) -> ()  [unwired: 10 in, 1 out]
          }
        }
        frame "SpliceIn" {
          w382 = u32 35  # Remove final frames
          w383 = 1000  # Splice ref
          w385 = 1250  # sub  unit real time
          # "This is start time of splice section. 1000x4 is 0.4s"
          # "This is time of 5000 frame processing chuck. 4x is 0.5s"
          # "Splice in New frames"
          n173 = Array Size(array=w388) -> (size(s)=w391:i32)
          n174 = Divide(x=w391, y=w390) -> (x/y=w389:dbl)
          n175 = Split 1D Array(array=w388, index=w389) -> (first subarray=w386:T12, second subarray=w387:T12)
          n176 = for {
            tunnel: w394 -> [w425]
            tunnel: w380 -> [w421]
            tunnel: w381 -> [w420]
            tunnel: w385 -> [w418]
            tunnel: "Splice" -> [w417]
            tunnel: w387 -> [w404] mode=indexing
            tunnel: w393 -> [w408]
            tunnel: w392 -> [w406]
            tunnel: w386 -> [w401] mode=indexing
            tunnel: w383 -> [w398]
            tunnel: w382 -> [w396]
            n177 = Add(x=w421, y=w420) -> (x+y=w419:i32)
            n178 = Unbundle By Name(w404) -> ("AVI Refnum"=w415:T5, "New Image"=w414:T1, "Number of Frames"=w416:u32)
            n179 = Add(x=w416, y=w417) -> (x+y=w397:u32)
            n180 = Subtract(x=w397, y=w396) -> (x-y=w395:u32)
            n181 = Unbundle By Name(w404) -> ("Frame Data"=w413:T8, "file name"=w400:string)
            n182 = Unbundle By Name(w401) -> ("AVI Refnum"=w403:T5, "New Image"=w402:T1)
            n183 = Concatenate Strings(w408, "Splice" ("string"), w400) -> (w409:string)
            n184 = local write "CurrentSaveFile"(w400) -> ()
            n185 = Unbundle By Name(w413) -> ("Frames Per Second"=w412:u32, "Codec"=w411:string)
            n186 = Build Path(base path=w406, name or relative path=w409) -> (appended path=w410:path)
            n187 = call "IMAQ AVI2 Create"("Codec"=w411, "Frames Per Second"=w412, "AVI Path"=w410) -> ("AVI Refnum"=w405:T5)  [unwired: 7 in, 1 out]
            n188 = for {
              N: w395 -> [_]
              tunnel: w425 -> [w445]
              tunnel: [w448] -> w424
              tunnel: [w447] -> w423
              tunnel: w405 -> [w446]
              tunnel: w402 -> [w444]
              tunnel: w403 -> [w443]
              tunnel: w420 -> [w437]
              tunnel: [w439] -> w422
              tunnel: w419 -> [w438]
              tunnel: w418 -> [w436]
              tunnel: w417 -> [w433]
              tunnel: w415 -> [w431]
              tunnel: w414 -> [w430]
              tunnel: [w427] -> w399 mode=indexing
              tunnel: w398 -> [w426]
              i -> [w434]
              n189 = Subtract(x=w434, y=w433) -> (x-y=w432:i32)
              n190 = Greater Or Equal?(x=w434, y=w436) -> (x >= y?=w435:bool)
              n191 = In Range and Coerce(upper limit=w438, x=w434, lower limit=w437) -> (In Range?=w440:bool)  [unwired: 1 out]
              n192 = Select(t=w432, s=w435, f=w434) -> (s? t:f=w428:i32)
              n193 = call "IMAQ AVI2 Read Frame"("error in (no error)"=w445, "Frame Number"=w428, "Image"=w430, "AVI Refnum"=w431) -> ("Image Out"=w442:T1, "AVI Refnum (duplicate)"=w447:T5)  [unwired: 5 in, 1 out]
              n194 = case shown="True" w440 {
                tunnel: w444 -> [_ w457]
                tunnel: w443 -> [w449 w456]
                tunnel: [w450 w455] -> w441
                tunnel: w442 -> [w450 _]
                tunnel: [w449 w454] -> w439
                tunnel: w434 -> [_ w453]
                tunnel: w426 -> [_ w452]
                tunnel: [_ w451] -> w429
                frame False {
                }
                frame True {
                  n195 = Subtract(x=w453, y=w452) -> (x-y=w451:i32)
                  n196 = call "IMAQ AVI2 Read Frame"("Frame Number"=w451, "Image"=w457, "AVI Refnum"=w456) -> ("Image Out"=w455:T1, "AVI Refnum (duplicate)"=w454:T5)  [unwired: 6 in, 1 out]
                }
              }
              n197 = Build Array(w428, w429) -> (w427:i32[])
              n198 = local write "Output"(w441) -> ()
              n199 = call "IMAQ AVI2 Write Frame"("Image"=w441, "AVI Refnum"=w446) -> ("AVI Refnum (duplicate)"=w448:T5)  [unwired: 7 in, 2 out]
              "Frame" <- w434
            }
            "Array 2" <- w399
            n200 = call "IMAQ AVI2 Close"("AVI Refnum"=w424) -> ()  [unwired: 10 in, 1 out]
            n201 = call "IMAQ AVI2 Close"("AVI Refnum"=w423) -> ()  [unwired: 10 in, 1 out]
            n202 = call "IMAQ AVI2 Close"("AVI Refnum"=w422) -> ()  [unwired: 10 in, 1 out]
          }
        }
      }
    }
  }
